vi "que_flush_and_wait_new_element.vi"(8 "error in (no error)":errorcluster, 11 "queue in":refnum<queue>) -> (0 "error out":errorcluster, 3 "queue out":refnum<queue>)   [LabVIEW 2013]
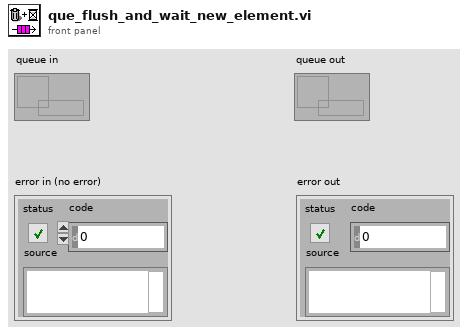
[diagram p1: front panel]
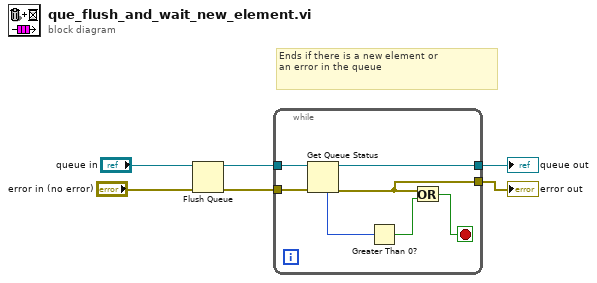
[diagram p0: block diagram]
diagram:
  # "Ends if there is a new element or\nan error in the queue"
  n1 = Flush Queue(queue="queue in", error in (no error)="error in (no error)") -> (queue out=w6:refnum<queue>, error out=w3:errorcluster)  [unwired: 1 out]
  n2 = while {
    tunnel: w6 -> [w13]
    tunnel: w3 -> [w11]
    tunnel: [w8] -> w2
    tunnel: [w7] -> w1
    stop <- w9 stop-if-true
    n3 = Get Queue Status(queue=w13, error in (no error)=w11) -> (queue out=w8:refnum<queue>, error out=w7:errorcluster, # elements in queue=w12:i32)  [unwired: 1 in, 5 out]
    n4 = Greater Than 0?(x=w12) -> (x > 0?=w10:bool)
    n5 = Or(x=w7, y=w10) -> (x .or. y?=w9:bool)
  }
  "queue out" <- w2
  "error out" <- w1
